vi "Write Test Case object to front panel control.vi"(8 "error in (no error)":errorcluster, 11 "LUnit Test Case In":refnum<class "LUnit Inheriting Test Case.lvclass">) -> (0 "error out":errorcluster, 3 "LUnit Test Case Out":refnum<class "LUnit Inheriting Test Case.lvclass">)   [LabVIEW 2020]
uses:
  LUnit Inheriting Test Case.lvclass
  C:/git/astemes-lunit/source/API/LUnit Test Case/LUnit Test Case.lvclass
  C:/git/astemes-lunit/source/Core/Runnable/Runnable.lvclass
  C:/git/astemes-lunit/source/API/LUnit Inheriting Test Case/LUnit Test Case/LUnit Inheriting Test Case.lvclass
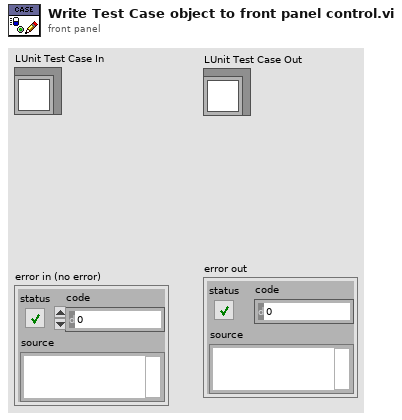
[diagram p1: front panel]
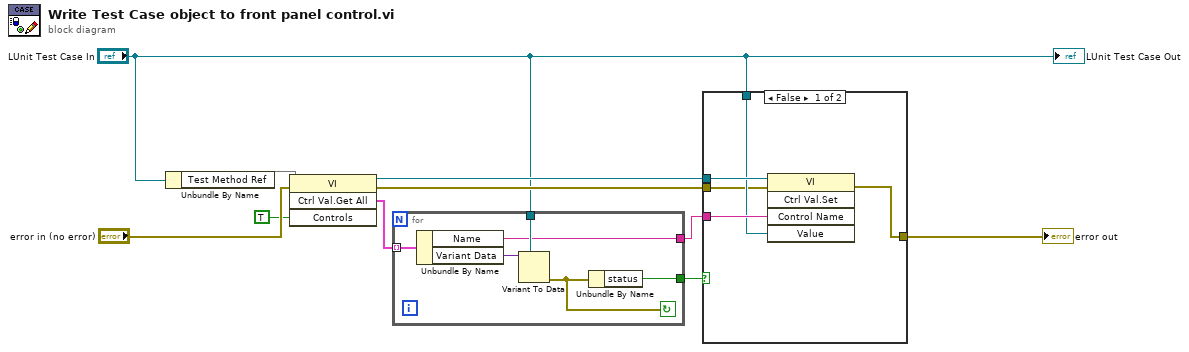
[diagram p0: block diagram]
diagram:
  n1 = Unbundle By Name("LUnit Test Case In") -> ("Test Method Ref"=w2)
  n2 = invoke on="Invoke Node" class="VI" method="Ctrl Val.Get All"(reference=w2, error in="error in (no error)", "Controls"=TRUE) -> (reference out=w4:refnum<vi>, error out=w9:errorcluster, "Get All Control Values Variant"=w6:cluster{"Name":string, "Variant Data":variant}[])  [unwired: 1 in, 1 out]
  n3 = for {
    tunnel: w6 -> [w16] mode=indexing
    tunnel: "LUnit Test Case In" -> [w14]
    tunnel: [w13] -> w7
    tunnel: [w11] -> w8
    stop <- w12 continue-if-true
    n4 = Unbundle By Name(w16) -> ("Name"=w13:string, "Variant Data"=w15:variant)
    n5 = Variant To Data(type=w14, Variant=w15) -> (error out=w12:errorcluster)  [unwired: 1 in, 1 out]
    n6 = Unbundle By Name(w12) -> ("status"=w11:bool)
  }
  n7 = case shown="False" w8 {
    tunnel: w4 -> [w21 _]
    tunnel: w7 -> [w20 _]
    tunnel: "LUnit Test Case In" -> [w19 _]
    tunnel: w9 -> [w18 w22]
    tunnel: [w17 w22] -> w3
    frame False {
      n8 = invoke on="Invoke Node" class="VI" method="Ctrl Val.Set"(reference=w21, error in=w18, "Control Name"=w20, "Value"=w19) -> (error out=w17:errorcluster)  [unwired: 1 in, 4 out]
    }
    frame True {
    }
  }
  "error out" <- w3
  "LUnit Test Case Out" <- "LUnit Test Case In"
